vi "Write Version string.vi"(10 "Version string":string, 11 "SolutionBuilder in":refnum<class "SolutionBuilder.lvclass">) -> (3 "SolutionBuilder out":refnum<class "SolutionBuilder.lvclass">)   [LabVIEW 2019, in "SolutionBuilder.lvlib" / "SolutionBuilder.lvclass"]
uses:
  SolutionBuilder.lvclass
  SolutionBuilder.lvclass/SolutionBuilder.ctl
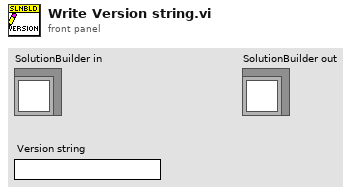
[diagram p1: front panel]
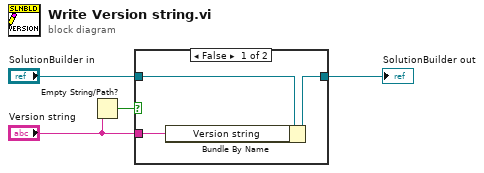
[diagram p0: block diagram]
diagram:
  n1 = Empty String/Path?(string/path="Version string") -> (empty?=w1:bool)
  n2 = case shown="False" w1 {
    tunnel: "SolutionBuilder in" -> [w7 w8]
    tunnel: [w6 w8] -> w3
    tunnel: "Version string" -> [w5 _]
    frame False {
      n3 = Bundle By Name(cluster=w7, "Version string"=w5) -> (w6:refnum<class "SolutionBuilder.lvclass">)
    }
    frame True {
    }
  }
  "SolutionBuilder out" <- w3
